vi "保存mes.vi"(7 "温度instance":refnum<class "Modbus Master.lvclass">, 11 "参数值":T1(array[cluster])) -> (2 "进站OK?":bool)   [LabVIEW 2020]
uses:
  <vilib>/NI/Modbus Library/API/Master/Modbus Master.lvclass
  Global.vi
  <vilib>/Utility/file.llb/Write Delimited Spreadsheet (string).vi
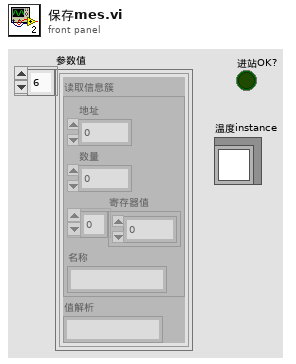
[diagram p1: front panel]
types:
  T1 = cluster{"读取信息簇":cluster{"地址":u16, "数量":u16, "寄存器值":u16[], "名称":string}, "值解析":string}[]
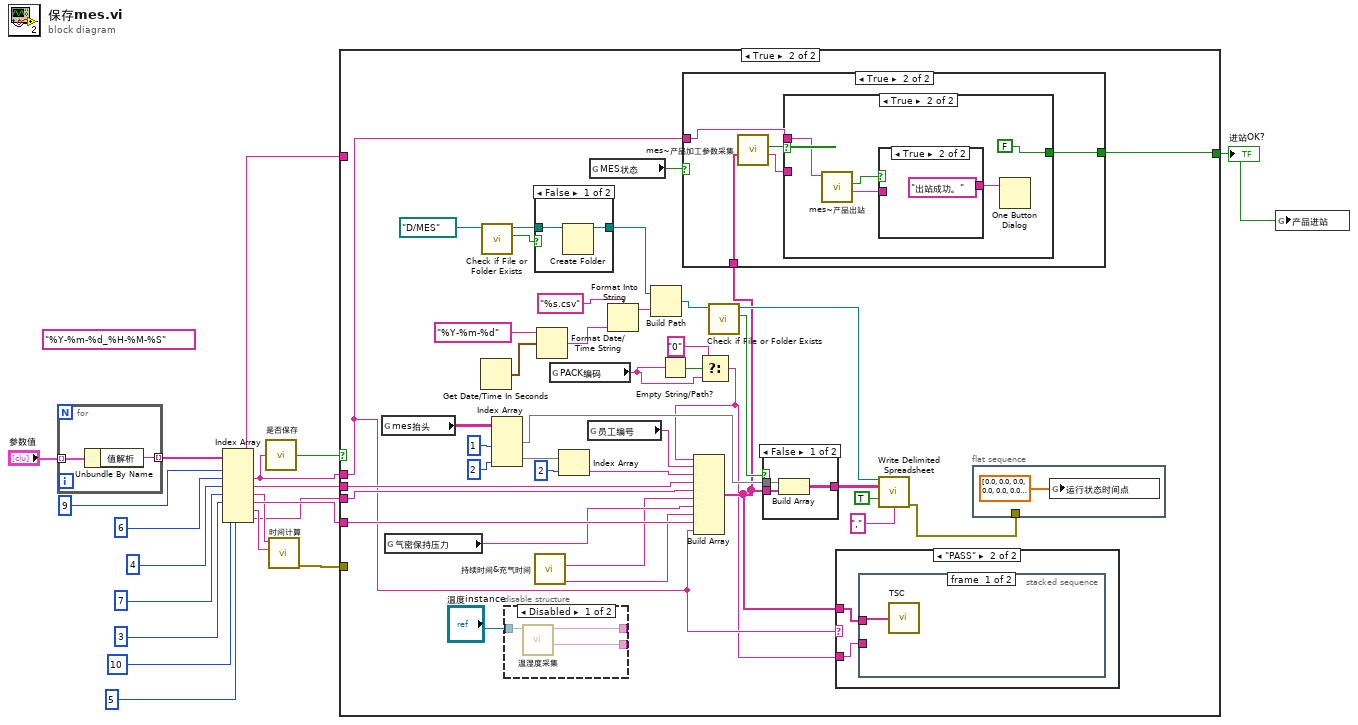
[diagram p0: block diagram]
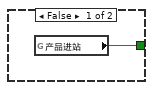
[diagram p2: hidden frame]
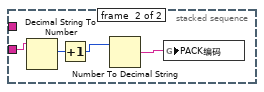
[diagram p4: hidden frame]
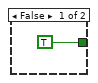
[diagram p6: hidden frame]
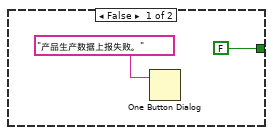
[diagram p7: hidden frame]
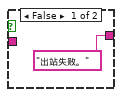
[diagram p8: hidden frame]
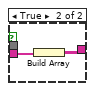
[diagram p9: hidden frame]
diagram:
  (unwired) "%Y-%m-%d_%H-%M-%S" ("时间格式字符串(%c)")
  n1 = for {
    tunnel: "参数值" -> [w21] mode=indexing
    tunnel: [w20] -> w18 mode=indexing
    n2 = Unbundle By Name(w21) -> ("值解析"=w20:string)
  }
  n3 = Index Array(array=w18, index #1=9 ("索引"), index #2=6 ("索引"), index #3=4 ("索引"), index #4=7 ("索引"), index #5=3 ("索引"), index #6=10 ("索引"), index #7=5 ("索引")) -> (element #1=w4:string, element #2=w13:string, element #3=w12:string, element #4=w8:string, element #5=w11:string, element #6=w7:string, element #7=w1:string)
  n4 = call "是否保存.vi"("测试结果"=w13) -> ("保存"=w10:bool)
  n5 = call "时间计算.vi"("运行状态"=w7, "实时压力"=w8) -> ("错误常量out"=w6:errorcluster)  [unwired: 9 in]
  n6 = case shown="True" w10 {
    tunnel: w13 -> [_ w27]
    tunnel: w12 -> [_ w49]
    tunnel: w1 -> [_ w48]
    tunnel: w11 -> [_ w47]
    tunnel: w6 -> [_ _]
    tunnel: w4 -> [_ _]
    tunnel: [w22 w31] -> w3
    frame False {
      n7 = global read "Global.vi" "产品进站"() -> (w22:bool)
    }
    frame True {
      n8 = global read "Global.vi" "mes抬头"() -> (w56:string[][])
      n9 = global read "Global.vi" "气密保持压力"() -> (w35:string)
      n10 = Get Date/Time In Seconds() -> (seconds since 1Jan1904=w60:timestamp)
      n11 = call <vilib>:"Check if File or Folder Exists.vi"("path"=path "D:/MES" ("路径")) -> ("file or folder exists?"=w43:bool, "dup path"=w42:path)  [unwired: 8 in, 1 out]
      n12 = Index Array(array=w56, index (col) #1=1 ("禁用的索引 (列)"), index (col) #2=2 ("禁用的索引 (列)")) -> (element #1=w46:string[], element #2=w53:string[])  [unwired: 2 in]
      n13 = disable-structure shown="Disabled" {
        disable-tunnel: "温度instance" -> [w71 _]
        disable-tunnel: [w70 _] -> _
        disable-tunnel: [w69 _] -> _
        frame Disabled {
          n14 = call "温湿度采集.vi"("Modbus Master输入"=w71) -> ("温度"=w69:string, "湿度"=w70:string)  [unwired: 9 in]
        }
        frame Enabled {
        }
      }
      n15 = case shown="False" w43 {
        tunnel: w42 -> [w94 w95]
        tunnel: [w93 w95] -> w39
        frame False {
          n16 = Create Folder(path (use dialog)=w94) -> (created path=w93:path)  [unwired: 2 in, 2 out]
        }
        frame True {
        }
      }
      n17 = call "持续时间&充气时间.vi"() -> ("气密保持压力持续时间"=w32:string, "气密充气时间"=w33:string)  [unwired: 10 in]
      n18 = Format Date/Time String(time format string (%c)="%Y-%m-%d" ("时间格式字符串(%c)"), seconds (now)=w60) -> (date/time string=w58:string)  [unwired: 1 in]
      n19 = global read "Global.vi" "PACK编码"() -> (w24:string)
      n20 = Index Array(array=w53, index=2 ("索引")) -> (element=w50:string)
      n21 = global read "Global.vi" "员工编号"() -> (w51:string)
      n22 = global read "Global.vi" "MES状态"() -> (w30:bool)
      n23 = Format Into String(format string="%s.csv" ("格式字符串"), w58) -> (resulting string=w57:string)  [unwired: 2 in, 1 out]
      n24 = Build Path(base path=w39, name or relative path=w57) -> (appended path=w38:path)
      n25 = Empty String/Path?(string/path=w24) -> (empty?=w26:bool)
      n26 = Select(t="0", s=w26, f=w24) -> (s? t:f=w23:string)
      n27 = Build Array(w23, w51, w50, w49, w48, w33, w35, w32, w47, w27) -> (w28:string[])
      n28 = case shown="True" w30 {
        tunnel: w27 -> [_ w77]
        tunnel: w28 -> [_ w76]
        tunnel: [TRUE w73] -> w31
        frame False {
        }
        frame True {
          n29 = call "mes~产品加工参数采集.vi"("采集项"=w76) -> ("ErrorMessage"=w74:string, "加工参数采集成功"=w75:bool)  [unwired: 8 in, 1 out]
          n30 = case shown="True" w75 {
            tunnel: w77 -> [_ w84]
            tunnel: w74 -> [_ _]
            tunnel: [FALSE FALSE] -> w73
            frame False {
              n31 = One Button Dialog(message="产品生产数据上报失败。") -> ()  [unwired: 1 in, 1 out]
            }
            frame True {
              n32 = call "mes~产品出站.vi"("测试结果"=w84) -> ("ErrorMessage"=w82:string, "出站成功"=w83:bool)  [unwired: 8 in, 1 out]
              n33 = case shown="True" w83 {
                tunnel: w82 -> [_ _]
                tunnel: ["出站失败。" "出站成功。"] -> w81
                frame False {
                }
                frame True {
                }
              }
              n34 = One Button Dialog(message=w81) -> ()  [unwired: 1 in, 1 out]
            }
          }
        }
      }
      n35 = call <vilib>:"Check if File or Folder Exists.vi"("path"=w38) -> ("file or folder exists?"=w37:bool, "dup path"=w36:path)  [unwired: 8 in, 1 out]
      n36 = case shown="False" w37 {
        tunnel: w46 -> [w90 _]
        tunnel: w28 -> [w89 w92]
        tunnel: [w88 w91] -> w45
        frame False {
          n37 = Build Array(w90, w89) -> (w88:string[][])
        }
        frame True {
          n38 = Build Array(w92) -> (w91:string[][])
        }
      }
      n39 = case shown="\"PASS\"" w27 {
        tunnel: w28 -> [_ w63]
        tunnel: w23 -> [_ w62]
        frame "NG", Default {
        }
        frame "PASS" {
          n40 = stacked-sequence {
            tunnel: w63 -> [w64 _]
            tunnel: w62 -> [_ w67]
            frame #0 {
              n41 = call "TSC.vi"("参数"=w64) -> ()
            }
            frame #1 {
              n42 = Decimal String To Number(string=w67) -> (number=w66:i32)  [unwired: 2 in, 1 out]
              n43 = Increment(x=w66) -> (x+1=w65:i32)
              n44 = Number To Decimal String(number=w65) -> (decimal integer string=w68:string)  [unwired: 1 in]
              n45 = global write "Global.vi" "PACK编码"(w68) -> ()
            }
          }
        }
      }
      n46 = call-poly <vilib>:"Write Delimited Spreadsheet.vi"("file path (dialog if empty)"=w36, "2D data"=w45, "append to file? (new file:F)"=TRUE ("append to file? (F)"), "delimiter (\\t)"="," ("delimiter (\\t)")) -> ("error out"=w34:errorcluster)  [unwired: 10 in, 1 out]
      n47 = flat-sequence {
        tunnel: w34 -> [_]
        frame #0 {
          n48 = global write "Global.vi" "运行状态时间点"(dbl[] [0.0, 0.0, 0.0, 0.0, 0.0, 0.0, 0.0, 0.0, 0.0] ("运行状态时间点")) -> ()
        }
      }
    }
  }
  "进站OK?" <- w3
  n49 = global write "Global.vi" "产品进站"(w3) -> ()
